vi "20T_Set_Setpoint.vi"() -> ()   [LabVIEW 2016]
uses:
  Equipment/Mercury iXX/Public/Controls/Mercury Reference.ctl
  Equipment/Mercury iXX/Public/Controls/Comms Transport Layer.ctl
  Equipment/Mercury iXX/Private/Controls/Query Dynamic Reference.ctl
  Utility/Monitor Communication/Gustav/20T_Cluster.ctl
  Equipment/Mercury iXX/Public/Libraries/Magnet/Open/Open Magnet Device.vi
  Equipment/Mercury iXX/Mercury iXX.lvlib
  Equipment/Mercury iXX/Public/Libraries/Magnet.lvlib
panel:
  in  "20T Control":T1={"Clamp"=TRUE, "Switch Heater"=TRUE, "Go to Zero"=TRUE, "Go to set"=FALSE, "Go to Hold"=FALSE, "Clamped"=FALSE, "Quenched"=FALSE, "Rate limit"=FALSE, "Persistent"=FALSE, "Hold"=FALSE, "Set"=FALSE, "Zero"=FALSE, "Magnet (T)"=0.0, "Leads (T)"=0.0, "Magnet T (K)"=3.4572, "Switch"=FALSE, "Target (T)"=3.4572, "Setpoint (T)"=0.0, "Rate (T/min)"=0.0, "Switch Heater 2"=FALSE, "Set Rate"=FALSE} {"Rate (T/min)" format="%6_5f"; "Setpoint (T)" format="%6_5f"; "Target (T)" format="%#4_5f"; "Magnet T (K)" format="%#4_5f"; "Leads (T)" format="%6_5f"}
  out "error out":errorcluster
  in  "Mercury Reference In":T2
  in  "error in (no error)":errorcluster
  # "20 T"
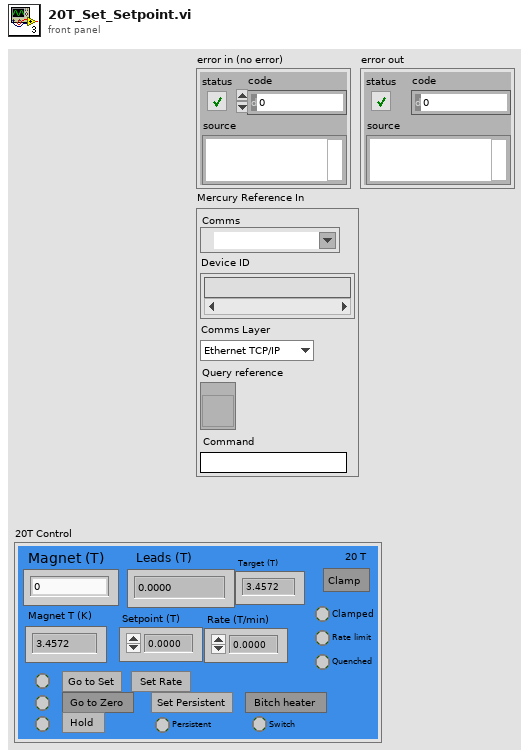
[diagram p1: front panel]
types:
  T1 = typedef "20T_Cluster.ctl" = cluster{"Clamp":bool, "Switch Heater":bool, "Go to Zero":bool, "Go to set":bool, "Go to Hold":bool, "Clamped":bool, "Quenched":bool, "Rate limit":bool, "Persistent":bool, "Hold":bool, "Set":bool, "Zero":bool, "Magnet (T)":dbl, "Leads (T)":dbl, "Magnet T (K)":dbl, "Switch":bool, "Target (T)":dbl, "Setpoint (T)":dbl, "Rate (T/min)":dbl, "Switch Heater 2":bool, "Set Rate":bool}
  T2 = typedef "Mercury iXX.lvlib/Mercury Reference.ctl" = cluster{"Comms":refnum<visa-resource-name>, "Device ID":string[], "Comms Layer":T3, "Command":string, "Query reference":T4}
  T3 = typedef "Mercury iXX.lvlib/Comms Transport Layer.ctl" = enum16{"Ethernet TCP/IP", "USB", "ISOBus - RS-232", "GPIB"}
  T4 = typedef "Mercury iXX.lvlib/Query Dynamic Reference.ctl" = refnum<vi>
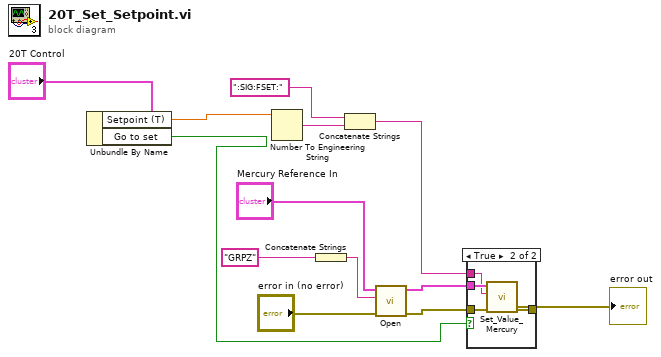
[diagram p0: block diagram]
diagram:
  n1 = Unbundle By Name("20T Control") -> ("Setpoint (T)"=w9:dbl, "Go to set"=w1:bool)
  n2 = Number To Engineering String(4:w9) -> (0:w10:string)  [unwired: 3 in]
  n3 = Concatenate Strings("GRPZ" ("Device Identifier")) -> (w7:string)
  n4 = Concatenate Strings(":SIG:FSET:", w10) -> (w6:string)
  n5 = call-poly "Open.vi"("error in (no error)"="error in (no error)", "Device Identifier"=w7, "Mercury Reference In"="Mercury Reference In") -> ("error out"=w11:errorcluster, "Mercury Reference Out"=w12:T2)  [unwired: 1 in, 6 out]
  n6 = case shown="True" w1 {
    tunnel: w12 -> [_ w18]
    tunnel: w11 -> [w14 w15]
    tunnel: [w14 w16] -> w4
    tunnel: w6 -> [_ w17]
    frame False {
    }
    frame True {
      n7 = call "Set_Value_Mercury.vi"("error in"=w15, "Noun(s)"=w17, "Mercury Reference In"=w18) -> ("error out"=w16:errorcluster)  [unwired: 7 in, 1 out]
    }
  }
  "error out" <- w4
